vi "Assignment _MechanicalAction.vi"() -> ()   [LabVIEW 2019]
panel:
  in  "stop":bool
  out "Counter":u16
  in  "Button":bool
  # "Button Mechanical Action"
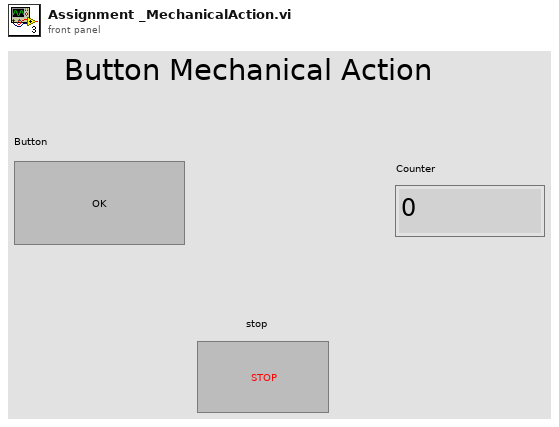
[diagram p1: front panel]
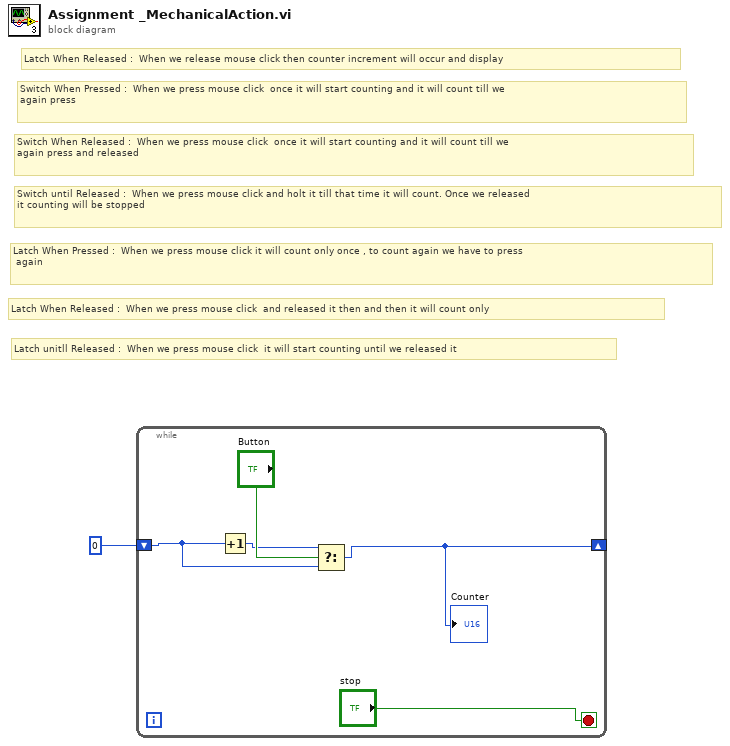
[diagram p0: block diagram]
diagram:
  # "Latch unitll Released :  When we press mouse click  it will start counting until we released it"
  # "Latch When Released :  When we press mouse click  and released it then and then it will count only"
  # "Latch When Pressed :  When we press mouse click it will count only once , to count again we have to press\n again"
  # "Switch until Released :  When we press mouse click and holt it till that time it will count. Once we released \nit counting will be stopped"
  # "Switch When Released :  When we press mouse click  once it will start counting and it will count till we\nagain press and released"
  # "Switch When Pressed :  When we press mouse click  once it will start counting and it will count till we\nagain press"
  # "Latch When Released :  When we release mouse click then counter increment will occur and display"
  n1 = while {
    shift-right: [w3] -> _
    shift-left: u16 0 ("Counter") -> [w4]
    stop <- "stop" stop-if-true
    n2 = Increment(x=w4) -> (x+1=w5:u16)
    n3 = Select(t=w5, s="Button", f=w4) -> (s? t:f=w3:u16)
    "Counter" <- w3
  }
